vi "File Open Logic.vi"(0 "PathIn":path=path "C:/ER2005/Data", 1 "Filename":string="Test001.txt", 6 "No Append":bool, 7 "Auto Append":bool, 8 "No Cancel":bool, 10 "No New":bool) -> (14 "FullPathOut":path, 15 "AppndOut":bool, 16 "ReplOut":bool, 17 "CancelOut":bool, 18 "NewOut":bool, 19 "ErrOut":bool)   [LabVIEW 2013]
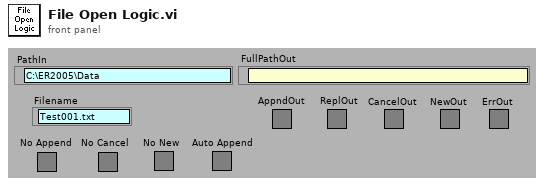
[diagram p1: front panel]
types:
  T1 = enum16{"open", "open or create", "create or replace", "create", "open (read only)"}
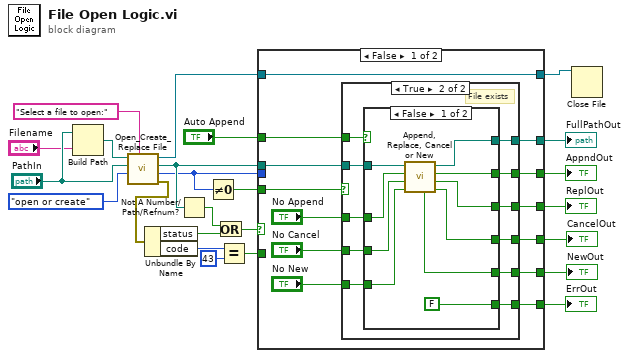
[diagram p0: block diagram]
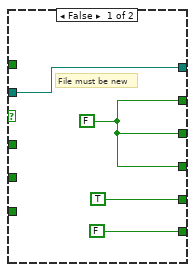
[diagram p2: hidden frame]
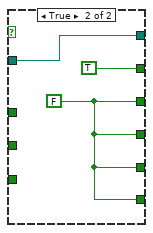
[diagram p3: hidden frame]
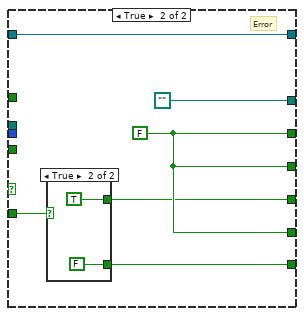
[diagram p4: hidden frame]
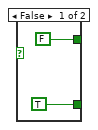
[diagram p5: hidden frame]
diagram:
  n1 = Build Path(base path="PathIn", name or relative path="Filename") -> (appended path=w20:path)
  n2 = call <vilib>:"Open_Create_Replace File.vi"("prompt"="Select a file to open:", "function (open:0)"=T1."open or create", "start path  (Not A Path)"="PathIn", "file path"=w20) -> ("error out"=w10:errorcluster, "file size (bytes)"=w9:i32, "new file path"=w13:path, "refnum"=w6:refnum<file>)  [unwired: 4 in]
  n3 = Unbundle By Name(w10) -> ("status"=w15:bool, "code"=w4:i32)
  n4 = Not A Number/Path/Refnum?(number/path/refnum=w13) -> (NaN/Path/Refnum?=w14:bool)
  n5 = Not Equal To 0?(x=w9) -> (x != 0?=w8:bool)
  n6 = Or(x=w14, y=w15) -> (x .or. y?=w5:bool)
  n7 = Equal?(x=w4, y=43) -> (x = y?=w2:bool)
  n8 = case shown="False" w5 {
    tunnel: w9 -> [_ _]
    tunnel: [w37 path ""] -> w19
    tunnel: w13 -> [w36 _]
    tunnel: [w35 w69] -> w18
    tunnel: [w34 w69] -> w17
    tunnel: [w33 w67] -> w16
    tunnel: [w32 w69] -> w12
    tunnel: [w31 w66] -> w11
    tunnel: w8 -> [w30 _]
    tunnel: [w29 w70] -> w7
    tunnel: w6 -> [w29 w70]
    tunnel: w2 -> [_ w68]
    tunnel: "Auto Append" -> [w25 _]
    frame False {
      n9 = case shown="True" w30 {
        tunnel: w36 -> [w41 w52]
        tunnel: [w41 w51] -> w37
        tunnel: [w40 w49] -> w35
        tunnel: [w40 w48] -> w34
        tunnel: [w40 w47] -> w33
        tunnel: [TRUE w46] -> w32
        tunnel: [FALSE w50] -> w31
        tunnel: "No Append" -> [_ w45]
        tunnel: "No Cancel" -> [_ w44]
        tunnel: "No New" -> [_ w43]
        tunnel: w25 -> [_ w42]
        frame False {
          w40 = FALSE ("AppndOut")
          # "File must be new"
        }
        frame True {
          # "File exists"
          n10 = case shown="False" w42 {
            tunnel: w52 -> [w62 w65]
            tunnel: [w61 w65] -> w51
            tunnel: [FALSE w63] -> w50
            tunnel: [w59 TRUE ("AppndOut")] -> w49
            tunnel: [w58 w63] -> w48
            tunnel: [w57 w63] -> w47
            tunnel: [w56 w63] -> w46
            tunnel: w45 -> [w55 _]
            tunnel: w44 -> [w54 _]
            tunnel: w43 -> [w53 _]
            frame False {
              n11 = call "Append, Replace, Cancel or New.vi"("NoNew"=w53, "NoCancel"=w54, "NoAppend"=w55, "PathIn"=w62) -> ("CancelOut"=w57:bool, "ReplOut"=w58:bool, "AppndOut"=w59:bool, "PathOut"=w61:path, "NewOut"=w56:bool)  [unwired: 3 in]
            }
            frame True {
              w63 = FALSE ("ReplOut")
            }
          }
        }
      }
    }
    frame True {
      w69 = FALSE
      # "Error"
      n12 = case shown="True" w68 {
        tunnel: [FALSE TRUE] -> w67
        tunnel: [TRUE FALSE] -> w66
        frame False {
        }
        frame True {
        }
      }
    }
  }
  "FullPathOut" <- w19
  "ReplOut" <- w17
  "AppndOut" <- w18
  "CancelOut" <- w16
  "NewOut" <- w12
  "ErrOut" <- w11
  n13 = Close File(refnum=w7) -> ()  [unwired: 1 in, 2 out]
